vi "Tuning.vi"() -> ()   [LabVIEW 2018]
uses:
  Type Defs/State Machine.ctl
  Type Defs/Open IPF.ctl
  <vilib>/Utility/config.llb/NI_LVConfig.lvlib
  <vilib>/Utility/config.llb/Read Key (Boolean).vi
  Type Defs/Global Action.ctl
  <vilib>/Utility/config.llb/Read Key (String).vi
  <vilib>/Utility/config.llb/Read Key (Path).vi
panel:
  in  "Run":bool
  out "XY Graph":cluster{"X":dbl, "Y":dbl}[](graph)
  in  "Tab":T1(tab)
  in  "Step vale":dbl
  in  "Stop Value":dbl
  in  "Start Value":dbl
  in  "Perform Parameter amp":bool
  in  "Ramping Parametrs":u8(ring)
  in  "Parameter Table":i32(listbox)
  in  "Error In":errorcluster
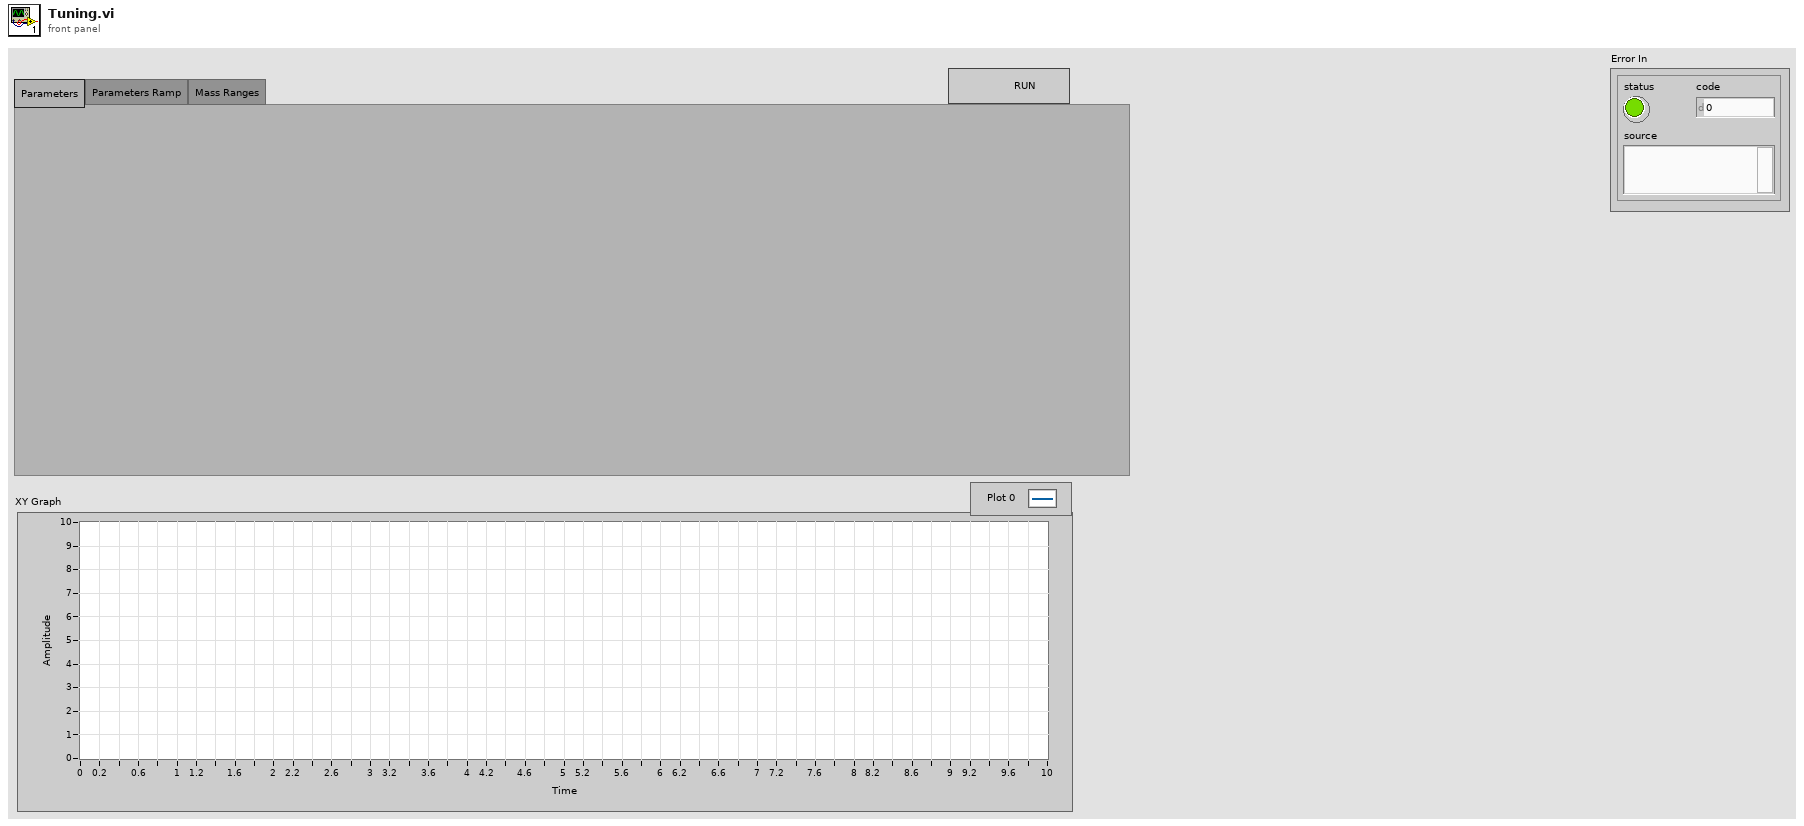
[diagram p1: front panel]
types:
  T1 = enum32{"Parameters", "Parameters Ramp", "Mass Ranges"}
  T2 = typedef "State Machine.ctl" = enum16{"Case 0", "Case 1", "Case 2", "Case 3", "Case 4", "Case 5", "Case 6", "Case 7", "Case 8", "Case 9", "Case 10", "Error", "Exit"}
  T3 = typedef "Global Action.ctl" = enum16{"Write", "Read"}
  T4 = typedef "Open IPF.ctl" = enum16{"Init", "Create IPF"}
  T5 = typedef "Global Parameters.ctl" = cluster{"Calibrations":cluster{"Q1 +ve":dbl[][], "Q2 +ve":dbl[][], "Q1 -ve":dbl[][], "Q2 -ve":dbl[][]}, "Resolution Q1":cluster{"High +ve":dbl[][], "Med +ve":dbl[][], "Low +ve":dbl[][], "High -ve":dbl[][], "Med -ve":dbl[][], "Low -ve":dbl[][]}, "Resolution Q2":cluster{"High +ve":dbl[][], "Med +ve":dbl[][], "Loe +ve":dbl[][], "High -ve":dbl[][], "Med -ve":dbl[][], "Low -ve":dbl[][]}, "MR Parameters":T6, "Mass":dbl[][], "Dwell":dbl[][], "Steps":i32[][], "Method Refnum":refnum<vi>}
  T6 = typedef "MR Parameters.ctl" = cluster{"Name":string, "Ch#":u8, "StartV":dbl, "StopV":dbl, "StepV":dbl, "Index":u8}
  T7 = typedef "NI_LVConfig.lvlib/Config Data RefNum.ctl" = refnum<k1>
  T8 = typedef "Global Configrations.ctl" = cluster{"Model Name":enum16{"QSight 110", "QSight 120", "QSight 210", "QSight 220", "QSight 410", "QSight 420", "IONICS 3Q 110", "IONICS 3Q 120", "IONICS 3Q 210", "IONICS 3Q 220", "IONICS 3Q 310", "IONICS 3Q 320", "Simulation (Single Source)", "Simulation (Dual Source)"}, "RunType":u16, "Acquisition State":enum16{"Ready", "Busy", "Waiting"}, "InstrState":enum16{"Initializing", "Mass Spectrometer is Off", "Starting Up", "Turning Power Off", "Going to Standby", "Roughing Pump Ready", "Turning Turbo Off", "Turbo Startup", "Turbopump Ready", "Checking Vacuum", "Going to Ready", "Ready", "Running", "Source Standby", "Lost Communication", "Shutting Down", "Fault", "24V Standby", "Go to 24V Standby", "Turbopump Ready-Waiting"}, "Run Mode":enum16{"MRM (Q1/Q2)", "Q1 Scan", "Q1 SRM", "Q2 Scan", "Q2 SRM", "Product Scan", "Precursor Scan", "Neutral Loss", "Neutral Gain"}, "Configration":T9, "TCP ID":refnum<k5>, "DT":bool, "Dead Time (nS)":i32, "Single Source":bool}
  T9 = typedef "Configration.ctl" = cluster{"Instrument":string[], "Tables":T10[]}
  T10 = typedef "Tables.ctl" = cluster{"Name":string, "Ch#":u8, "Min":dbl, "Max":dbl, "Def+":dbl, "Def-":dbl, "Offset":dbl, "Slope":dbl, "Type":u8, "Description":string, "SettleT":dbl}
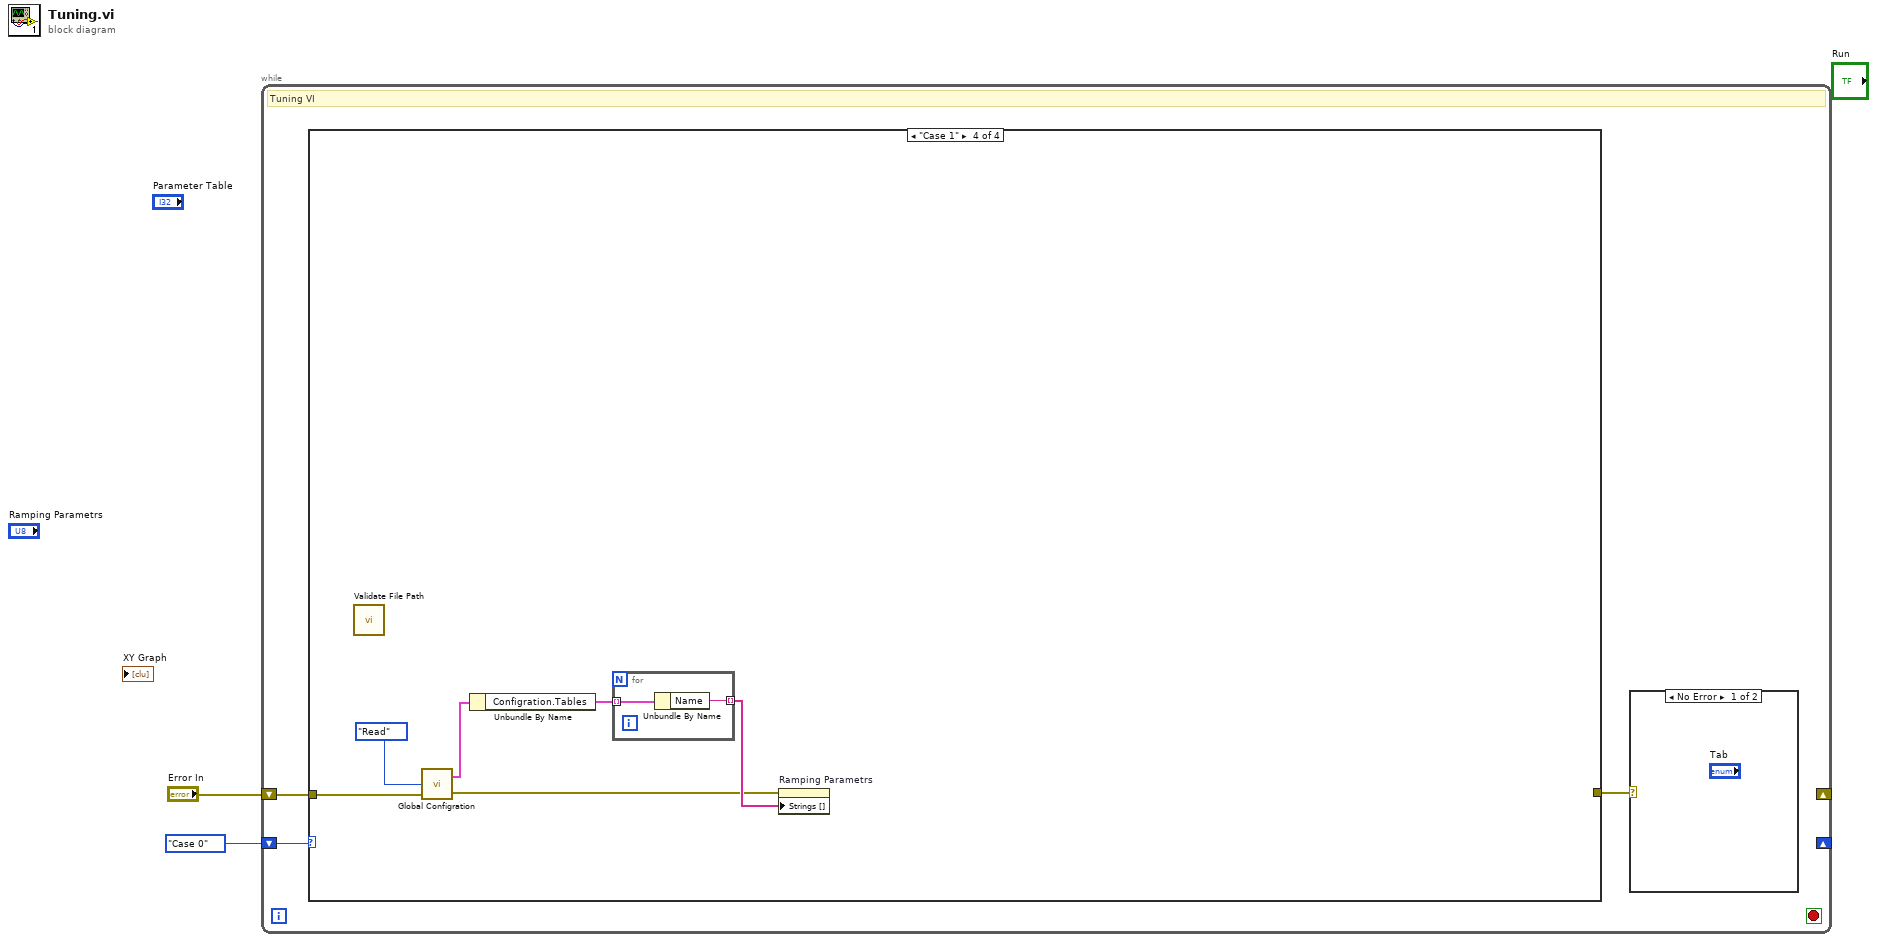
[diagram p0: block diagram]
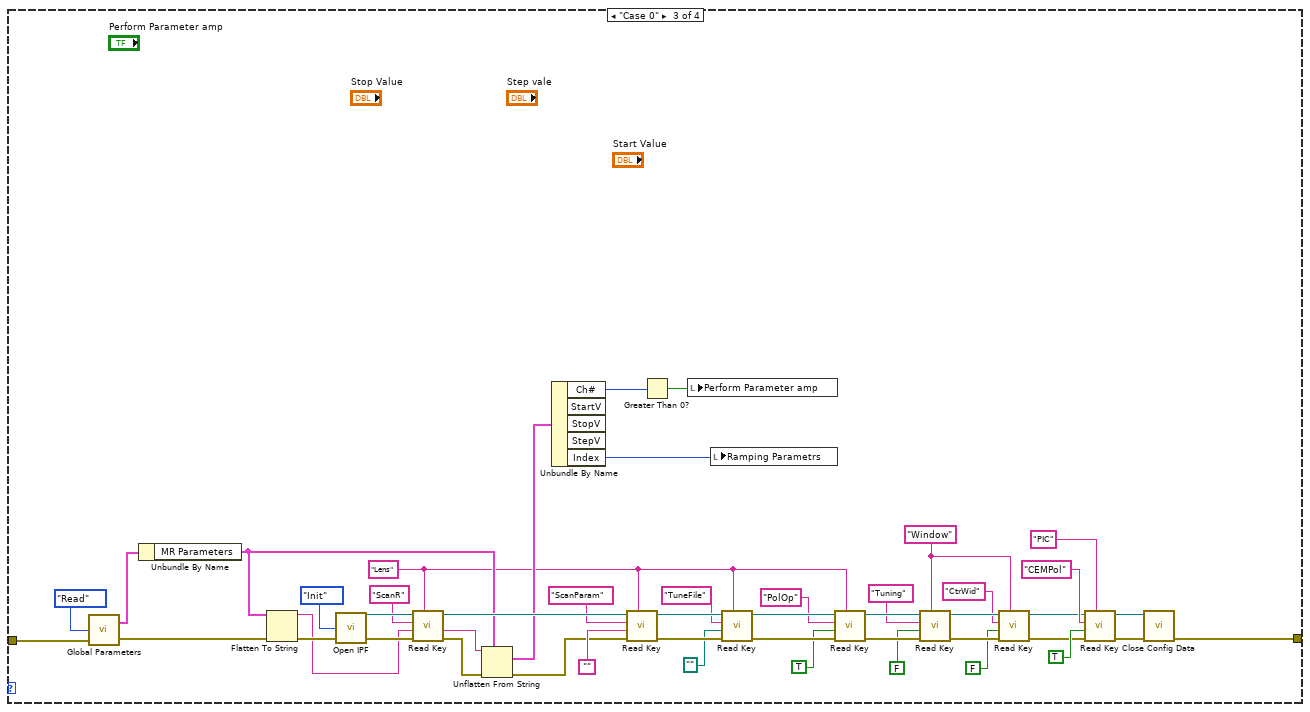
[diagram p4: hidden frame]
diagram:
  n1 = while {
    shift-right: _ -> [_]
    shift-left: "Error In" -> [w4]
    shift-right: _ -> [_]
    shift-left: State_Machine."Case 0" ("Enum") -> [w5]
    stop <- _ stop-if-true
    # "Tuning VI"
    n2 = case shown="\"Case 1\"" w5 {
      tunnel: w4 -> [_ _ w34 w58]
      tunnel: [_ _ w7 _] -> w3
      frame "Error", Default {
      }
      frame "Exit" {
      }
      frame "Case 0" {
        w12 = "Window" ("section")
        w18 = "Lens" ("section")
        n3 = call "Global Parameters.vi"("Error In"=w34, "Action"=Global_Action."Read") -> ("Error Out"=w28:errorcluster, "Parameters Out"=w32:T5)  [unwired: 1 in]
        n4 = Unbundle By Name(w32) -> ("MR Parameters"=w27:T6)
        n5 = Flatten To String(anything=w27, error in (no error)=w28) -> (data string=w30:string, error out=w31:errorcluster)  [unwired: 3 out]
        n6 = call "Open IPF.vi"("Error In"=w31, 4:Open_IPF."Init") -> ("Error Out"=w51:errorcluster, "IPF refnum"=w50:T7)  [unwired: 1 in, 1 out]
        n7 = call-poly <vilib>:"Read Key.vi"("section"=w18, "error in (no error)"=w51, "default value"=w30, "key"="ScanR" ("section"), "refnum"=w50) -> ("error out"=w25:errorcluster, "value"=w26:string, "refnum out"=w45:T7)  [unwired: 1 in, 3 out]
        n8 = Unflatten From String(type=w27, binary string=w26, error in (no error)=w25) -> (value=w24:T6, error out=w23:errorcluster)  [unwired: 3 out]
        n9 = Unbundle By Name(w24) -> ("Ch#"=w21:u8, "Index"=w6:u8)  [unwired: 3 out]
        n10 = call-poly <vilib>:"Read Key.vi"("section"=w18, "error in (no error)"=w23, "default value"="", "key"="ScanParam", "refnum"=w45) -> ("error out"=w49:errorcluster, "refnum out"=w44:T7)  [unwired: 1 in, 4 out]
        n11 = Greater Than 0?(x=w21) -> (x > 0?=w22:bool)
        n12 = local write "Perform Parameter amp"(w22) -> ()
        n13 = local write "Ramping Parametrs"(w6) -> ()
        n14 = call-poly <vilib>:"Read Key.vi"("section"=w18, "error in (no error)"=w49, "default value"=path "", "key"="TuneFile", "refnum"=w44) -> ("error out"=w48:errorcluster, "refnum out"=w43:T7)  [unwired: 5 out]
        n15 = call-poly <vilib>:"Read Key.vi"("section"=w18, "error in (no error)"=w48, "default value"=TRUE, "key"="PolOp" ("section"), "refnum"=w43) -> ("error out"=w47:errorcluster, "refnum out"=w42:T7)  [unwired: 5 out]
        n16 = call-poly <vilib>:"Read Key.vi"("section"=w12, "error in (no error)"=w47, "default value"=FALSE, "key"="Tuning" ("section"), "refnum"=w42) -> ("error out"=w13:errorcluster, "refnum out"=w14:T7)  [unwired: 5 out]
        n17 = call-poly <vilib>:"Read Key.vi"("section"=w12, "error in (no error)"=w13, "default value"=FALSE, "key"="CtrWid", "refnum"=w14) -> ("error out"=w9:errorcluster, "refnum out"=w8:T7)  [unwired: 5 out]
        n18 = call-poly <vilib>:"Read Key.vi"("section"="PIC", "error in (no error)"=w9, "default value"=TRUE, "key"="CEMPol" ("section"), "refnum"=w8) -> ("error out"=w46:errorcluster, "refnum out"=w41:T7)  [unwired: 5 out]
        n19 = call <vilib>:"Close Config Data.vi"("error in (no error)"=w46, "refnum"=w41) -> ("error out"=w7:errorcluster)  [unwired: 8 in, 1 out]
      }
      frame "Case 1" {
        n20 = call "Validate File Path.vi"() -> ()  [unwired: 5 in, 2 out]
        n21 = call "Global Configration.vi"("Error In"=w58, "Action"=Global_Action."Read") -> ("Error Out"=w54:errorcluster, "Parameters Out"=w57:T8)  [unwired: 1 in]
        n22 = Unbundle By Name(w57) -> ("Configration.Tables"=w56:T10[])
        n23 = for {
          tunnel: w56 -> [w60] mode=indexing
          tunnel: [w59] -> w55 mode=indexing
          n24 = Unbundle By Name(w60) -> ("Name"=w59:string)
        }
        n25 = property on="Ramping Parametrs" class="Ring (strict)"(error in=w54, "Strings []"=w55) -> ()  [unwired: 1 in, 2 out]
      }
    }
    n26 = case shown="No Error" w3 {
      frame No Error {
      }
      frame Error {
      }
    }
  }
